vi "UHR-Fleezers Control (host) -Leonardo 04-2018 V4_fish.vi"(0 "Tab Green FB":T5(tab)=enum."Trap Control (RF)") -> ()   [LabVIEW 2014] (continued)
                n1375 = Divide "Y V/pix"(x=w2136, y=w2151) -> (x/y=w2150:dbl)
                n1376 = Divide "Y half step offset"(x=w2136, y=2.0) -> (x/y=w2152:dbl)
                n1377 = Divide "X pix/step"(x=w2140, y=w2143) -> (x/y=w2149:dbl)
                n1378 = Negate(x=w2152) -> (-x=w2153:dbl)
                n1379 = local read "Initial Y"() -> (w2159:dbl)
                n1380 = Multiply(x=w2141, y=w2150) -> (x*y=w2160:dbl)
                n1381 = Divide "X half step offset"(x=w2136, y=2.0) -> (x/y=w2146:dbl)
                n1382 = Divide "X V/pix"(x=w2136, y=w2149) -> (x/y=w2148:dbl)
                n1383 = Multiply(x=w2136, y=w2143) -> (x*y=w2155:dbl)
                n1384 = Compound Arithmetic op=ADD(w2153, w2160, w2159) -> (w2137:dbl)
                "Pointer Y (V)" <- w2137
                n1385 = Multiply(x=w2148, y=w2142) -> (x*y=w2157:dbl)
                n1386 = Negate(x=w2146) -> (-x=w2145:dbl)
                n1387 = local read "Initial X"() -> (w2158:dbl)
                n1388 = Negate(x=w2157) -> (-x=w2156:dbl)
                n1389 = Compound Arithmetic op=ADD(w2145, w2155, w2158, w2156) -> (w2138:dbl)
                "Pointer X (V)" <- w2138
                n1390 = Or(x="Set X Only", y="Set Confocal Spot (X-Y)") -> (x .or. y?=w2131:bool)
                n1391 = Or(x="Set Confocal Spot (X-Y)", y="Set Y Only") -> (x .or. y?=w2130:bool)
                n1392 = case shown="True" w2131 {
                  tunnel: w2138 -> [_ w2161]
                  frame False {
                  }
                  frame True {
                    n1393 = property on="AO2" class="Slide (strict)"("Val(Sgnl)"=w2161) -> ()  [unwired: 2 in, 2 out]
                  }
                }
                n1394 = case shown="True" w2130 {
                  tunnel: w2137 -> [_ w2162]
                  frame False {
                  }
                  frame True {
                    n1395 = property on="AO1" class="Slide (strict)"("Val(Sgnl)"=w2162) -> ()  [unwired: 2 in, 2 out]
                  }
                }
                n1396 = local write "Set Confocal Spot (X-Y)"(w2135) -> ()
                n1397 = local write "Set X Only"(w2135) -> ()
                n1398 = local write "Set Y Only"(w2135) -> ()
              }
            }
          }
          frame 3 {
            n1399 = local read "BD 2 Frequency 1 (MHz)"() -> (w2163:dbl)
            n1400 = local read "BD 1 Frequency 1 (MHz)"() -> (w2164:dbl)
            n1401 = local write "Manipulating Trap"(TRUE ("Manipulating Trap")) -> ()
            n1402 = local write "Coords"(T8 {"Horizontal"=0, "Vertical"=0} ("Coords")) -> ()
            n1403 = while {
              tunnel: w2169 -> [w2174]
              tunnel: w2167 -> [w2173]
              tunnel: w2165 -> [w2172]
              tunnel: w2164 -> [w2171]
              tunnel: w2163 -> [w2170]
              stop <- w2175 stop-if-true
              n1404 = event shown="[0] \"Pane\": Mouse Move" {
                selector: _ -> [_ _]
                dyn-events: _ -> [_ _]
                timeout: _ -> [_ _]
                tunnel: ["Force Manip Abort" w2239] -> w2175
                tunnel: w2174 -> [w2182 _]
                tunnel: w2173 -> [w2180 _]
                tunnel: w2172 -> [w2179 _]
                tunnel: w2171 -> [w2178 _]
                tunnel: w2170 -> [w2177 _]
                event Mouse Move {
                  n1405 = event-data() -> ("Time"=w2183:u32, "Coords"=w2184:T8)  [unwired: 3 out]
                  n1406 = Less?(x=w2183, y=w2182) -> (x < y?=w2181:bool)
                  n1407 = case "Makes sure old motion events prior to mouse click aren't used" shown="False" w2181 {
                    tunnel: w2184 -> [w2226 _]
                    tunnel: w2180 -> [w2227 _]
                    tunnel: w2179 -> [w2204 _]
                    tunnel: w2178 -> [w2200 _]
                    tunnel: w2177 -> [w2199 _]
                    frame False {
                      n1408 = Subtract(x=w2226, y=w2227) -> (x-y=w2225:T8)
                      "Coords" <- w2225
                      n1409 = local read "Y RF Frequency Limits (MHz)"() -> (w2185:T16)
                      n1410 = To Double Precision Float(number=w2225) -> (double precision float=w2224:cluster{"Horizontal":dbl, "Vertical":dbl})
                      n1411 = Multiply(x=cluster{"Horizontal":dbl, "Vertical":dbl} {"Horizontal"=-1.0, "Vertical"=1.0}, y="Manipulation Scaling") -> (x*y=w2220:cluster{"Horizontal":dbl, "Vertical":dbl})
                      n1412 = local read "X RF Frequency Limits (MHz)"() -> (w2186:T16)
                      n1413 = Multiply(x=w2224, y=w2220) -> (x*y=w2222:cluster{"Horizontal":dbl, "Vertical":dbl})
                      n1414 = Unbundle By Name(w2222) -> ("Horizontal"=w2217:dbl, "Vertical"=w2221:dbl)
                      n1415 = Unbundle By Name(w2185) -> ("Maximum"=w2188:dbl, "Minimum"=w2187:dbl)
                      n1416 = Boolean To (0,1)(Boolean="Manip. X?") -> (0, 1=w2215:i16)
                      n1417 = Boolean To (0,1)(Boolean="Manip. Y?") -> (0, 1=w2212:i16)
                      n1418 = local read "BD 1 Frequency 2 (MHz)"() -> (w2202:dbl)
                      n1419 = Multiply(x=w2221, y=w2212) -> (x*y=w2214:dbl)
                      n1420 = Multiply(x=w2215, y=w2217) -> (x*y=w2218:dbl)
                      n1421 = local read "BD 2 Frequency 2 (MHz)"() -> (w2201:dbl)
                      n1422 = Unbundle By Name(w2186) -> ("Maximum"=w2190:dbl, "Minimum"=w2189:dbl)
                      n1423 = Add(x=w2199, y=w2214) -> (x+y=w2192:dbl)
                      n1424 = Add(x=w2200, y=w2218) -> (x+y=w2194:dbl)
                      n1425 = In Range and Coerce(upper limit=w2190, x=w2194, lower limit=w2189) -> (coerced(x)=w2193:dbl)  [unwired: 1 out]
                      n1426 = In Range and Coerce(upper limit=w2188, x=w2192, lower limit=w2187) -> (coerced(x)=w2191:dbl)  [unwired: 1 out]
                      n1427 = Subtract(x=w2193, y=w2202) -> (x-y=w2211:dbl)
                      n1428 = Subtract(x=w2191, y=w2201) -> (x-y=w2210:dbl)
                      n1429 = Square(x=w2211) -> (x^2=w2209:dbl)
                      n1430 = Square(x=w2210) -> (x^2=w2208:dbl)
                      n1431 = Add(x=w2209, y=w2208) -> (x+y=w2207:dbl)
                      n1432 = Square Root(x=w2207) -> (sqrt(x)=w2203:dbl)
                      n1433 = In Range and Coerce(upper limit="Limit Max (MHz)", x=w2203, lower limit="Limit Min (MHz)") -> (In Range?=w2196:bool)  [unwired: 1 out]
                      n1434 = Not(x="Limits Enable") -> (.not. x?=w2195:bool)
                      n1435 = Or(x=w2196, y=w2195) -> (x .or. y?=w2197:bool)
                      n1436 = case shown="True" w2197 {
                        tunnel: w2204 -> [_ w2237]
                        tunnel: w2203 -> [_ w2228]
                        tunnel: w2193 -> [_ w2235]
                        tunnel: w2202 -> [_ w2234]
                        tunnel: w2191 -> [_ w2233]
                        tunnel: w2201 -> [_ w2232]
                        tunnel: w2186 -> [_ w2230]
                        tunnel: w2185 -> [_ w2229]
                        frame False {
                        }
                        frame True {
                          n1437 = local read "BD 1 Frequency 3 (MHz)"() -> (w2236:dbl)
                          n1438 = local read "BD 2 Frequency 3 (MHz)"() -> (w2231:dbl)
                          n1439 = local write "Trap Delta (MHz)"(w2228) -> ()
                          n1440 = property on="Initial delta (MHz)" class="DigNum (strict)"("Val(Sgnl)"=w2228) -> ()  [unwired: 2 in, 2 out]
                          n1441 = call "set RF board frequency - interlace.vi"("Board 2 Frequency Limits"=w2229, "Board 1 Frequency Limits"=w2230, "FPGA VI Reference In"=w2237, "Board 2 Frequency 3 (MHz)"=w2231, "Board 1 Frequency 3 (MHz)"=w2236, "Board 2 Frequency 2 (MHz)"=w2232, "Board 2 Frequency 1 (MHz)"=w2233, "Board 1 Frequency 2 (MHz)"=w2234, "Board 1 Frequency 1  (MHz)"=w2235) -> ()  [unwired: 1 in, 2 out]
                          n1442 = local write "BD 2 Frequency 1 (MHz)"(w2233) -> ()
                          n1443 = local write "BD 1 Frequency 1 (MHz)"(w2235) -> ()
                        }
                      }
                    }
                    frame True {
                    }
                  }
                }
                event Mouse Up {
                  n1444 = event-data() -> ("Button"=w2238:u16)  [unwired: 8 out]
                  n1445 = case shown="3" w2238 {
                    tunnel: [FALSE TRUE] -> w2239
                    frame 0, Default {
                    }
                    frame 3 {
                      n1446 = local write "Manipulating Trap"(FALSE ("Manipulating Trap")) -> ()
                    }
                  }
                }
              }
            }
          }
        }
      }
      event Mouse Move {
        n1447 = event-data() -> ()  [unwired: 6 out]
      }
    }
    n1448 = local read "Stop All"() -> (w2060:bool)
    n1449 = node-c288() -> ()  [unwired: 2 out]
  }
  n1450 = node-c288(w54) -> ()  [unwired: 1 out]
  n1451 = node-c288(w103) -> ()  [unwired: 1 out]
  n1452 = node-c288(w110) -> ()  [unwired: 1 out]
  n1453 = node-c288(i64 1 ("Period"), 1 ("Processor")) -> (w196:T25)  [unwired: 2 out]
  n1454 = timed-loop "Acquire Data" {
    tunnel: w62 -> [w2550]
    tunnel: w77 -> [w2549]
    tunnel: [w2580] -> w70
    tunnel: [w2574] -> w3
    timing: w196 -> [_]
    timing-out: [_] -> w195
    tunnel: w94 -> [w2396]
    stop <- "Stop All" stop-if-true
    (unwired) u32 0 ("Number of Elements")
    w2383 = "NI_ChannelName" ("name")
    n1455 = node-c288() -> ()  [unwired: 2 out]
    n1456 = First Call?() -> (First Call?: T/F=w2349:bool)
    n1457 = Or(x="Reset", y=w2349) -> (x .or. y?=w2350:bool)
    n1458 = local read "MCL Tracking"() -> (w2287:bool)
    n1459 = case "Reset data stream" shown="True" w2350 {
      tunnel: w2550 -> [w2748 w2756]
      tunnel: w2549 -> [w2747 w2755]
      tunnel: [w2748 w2750] -> w2285
      tunnel: [w2747 w2749] -> w2545
      frame False {
      }
      frame True {
        w2753 = TRUE ("AI to FIFO")
        n1460 = local write "Overflow (data lost)"(FALSE ("Overflow (data lost)")) -> ()
        n1461 = call "reset FPGA DMA.vi"("error in"=w2755, "FPGA VI Reference In"=w2756) -> ("error out"=w2751:errorcluster, "FPGA VI Reference Out"=w2752:T20)
        n1462 = xnode "Read/Write Control"("FPGA VI Reference In"=w2752, "error in"=w2751, "AI to FIFO"=w2753, "APD to FIFO"=w2753) -> ("FPGA VI Reference Out"=w2750:T20, "error out"=w2749:errorcluster)
      }
    }
    n1463 = Or(x="Start AOD Scan", y="Trap Raster Scan") -> (x .or. y?=w2503:bool)
    n1464 = case "Start AOM raster scan" shown="True" w2503 {
      tunnel: w2285 -> [w3489 w3500]
      tunnel: w2545 -> [w3488 w3499]
      tunnel: [w3489 w3493] -> w2284
      tunnel: [w3488 w3492] -> w2544
      frame False {
      }
      frame True {
        n1465 = case shown="True" "Restart DMA? (AOD)" {
          tunnel: [w3540 w3542] -> w3494
          tunnel: [w3539 w3541] -> w3495
          tunnel: w3500 -> [w3540 w3544]
          tunnel: w3499 -> [w3539 w3543]
          frame False {
          }
          frame True {
            n1466 = local write "Overflow (data lost)"(FALSE ("Overflow (data lost)")) -> ()
            n1467 = call "reset FPGA DMA.vi"("error in"=w3543, "FPGA VI Reference In"=w3544) -> ("error out"=w3541:errorcluster, "FPGA VI Reference Out"=w3542:T20)
          }
        }
        n1468 = local write "Trap Raster Scan"(FALSE ("Trap Raster Scan")) -> ()
        n1469 = case shown="False" "Move MCL Also?" {
          tunnel: w3495 -> [w3504 w3534]
          tunnel: w3494 -> [w3505 w3535]
          tunnel: [w3503 w3538] -> w3493
          tunnel: [w3502 w3537] -> w3492
          tunnel: "Raster to target force?" -> [w3501 w3507]
          frame False {
            w3506 = TRUE ("AI to FIFO")
            n1470 = xnode "Read/Write Control"("FPGA VI Reference In"=w3505, "error in"=w3504, "AI to FIFO"=w3506, "APD to FIFO"=w3506, "Start scan"=w3506, "Raster to target force"=w3501) -> ("FPGA VI Reference Out"=w3503:T20, "error out"=w3502:errorcluster)
          }
          frame True {
            w3531 = FALSE ("1D or 2D Scan?")
            w3536 = TRUE ("AI to FIFO")
            # "Count for MCL loop"
            # "N total cycles"
            # "N steps"
            # "V_int"
            n1471 = local read "Scan Range (nm)"() -> (w3513:dbl)
            n1472 = local read "Number of F/B Scans (AOD)"() -> (w3530:u16)
            n1473 = Sign(1:w3513) -> (0:w3512:dbl)
            n1474 = Compound Arithmetic op=MULTIPLY(w3513, "MCL Step Position Ratio", "MCL/AOM Scale Tweak") -> (w3517:dbl)
            n1475 = Negate(x=w3512) -> (-x=w3509:dbl)
            n1476 = Multiply(x=w3509, y="MCL Step Increment (V_int)") -> (x*y=w3511:dbl)
            n1477 = Divide(x=w3517, y="MCL X Cal (nm/V)") -> (x/y=w3523:dbl)
            n1478 = Multiply(x=32767.0 ("y"), y=w3523) -> (x*y=w3529:dbl)
            n1479 = local read "Total Counts (ticks)"() -> (w3514:u32)
            n1480 = local read "Cycles/step (AOD)"() -> (w3525:u64)
            n1481 = local read "Scan steps (AOD)"() -> (w3526:u64)
            n1482 = Divide(x=w3529, y=10.0) -> (x/y=w3522:dbl)
            n1483 = Divide(x=w3522, y="MCL Step Increment (V_int)") -> (x/y=w3520:dbl)
            n1484 = Absolute Value(x=w3520) -> (abs(x)=w3508:dbl)
            n1485 = Compound Arithmetic op=MULTIPLY(w3526, w3525, w3514) -> (w3521:u64)
            n1486 = local write "wait to reset values"(w3536) -> ()
            n1487 = local write "MCL Scanning"(w3536) -> ()
            n1488 = Divide(x=w3521, y=w3508) -> (x/y=w3518:dbl)
            "MCL Count" <- w3518
            n1489 = xnode "Read/Write Control"("FPGA VI Reference In"=w3535, "error in"=w3534, "Scan steps (MCL)"=w3508, "Number of scans (MCL)"=w3530, "Cycles per step (MCL)"=u64 1, "Scan freq.  increment (MCL)"=w3511, "1D or 2D Scan?"=w3531, "MCL Scan Axis"=w3531, "Cont. Scan (MCL)"=w3531, "MCL count"=w3518) -> ("FPGA VI Reference Out"=w3533:T20, "error out"=w3532:errorcluster)
            n1490 = xnode "Read/Write Control"("FPGA VI Reference In"=w3533, "error in"=w3532, "AI to FIFO"=w3536, "APD to FIFO"=w3536, "Start scan"=w3536, "Start scan (MCL)"=w3536, "Raster to target force"=w3507) -> ("FPGA VI Reference Out"=w3538:T20, "error out"=w3537:errorcluster)
          }
        }
        "Raster Scanning..." <- TRUE ("Scanning...")
      }
    }
    n1491 = And(x="Save scans", y=w2503) -> (x .and. y?=w2543:bool)
    n1492 = Compound Arithmetic op=OR("Start MCL Scan", "Confocal Image", "Confocal Linescan") -> (w2501:bool)
    n1493 = And(x="Save Data (MCL)", y=w2501) -> (x .and. y?=w2542:bool)
    n1494 = case "Start MCL raster scan" shown="True" w2501 {
      tunnel: w2284 -> [w3039 w3054]
      tunnel: w2544 -> [w3038 w3053]
      tunnel: [w3039 w3049] -> w2319
      tunnel: [w3038 w3048] -> w2318
      tunnel: [FALSE w3047] -> w2528
      tunnel: "Start MCL Scan" -> [_ w3042]
      tunnel: "Confocal Image" -> [_ w3041]
      tunnel: "Confocal Linescan" -> [_ _]
      frame False {
      }
      frame True {
        w3047 = TRUE
        n1495 = case shown="True" "Restart DMA? (MCL)" {
          tunnel: [w3099 w3101] -> w3052
          tunnel: [w3098 w3100] -> w3051
          tunnel: w3054 -> [w3099 w3104]
          tunnel: w3053 -> [w3098 w3103]
          frame False {
          }
          frame True {
            n1496 = call "reset FPGA DMA.vi"("error in"=w3103, "FPGA VI Reference In"=w3104) -> ("error out"=w3100:errorcluster, "FPGA VI Reference Out"=w3101:T20)
            n1497 = local write "Overflow (data lost)"(FALSE ("Overflow (data lost)")) -> ()
          }
        }
        n1498 = case shown="False" w3042 {
          selector: w3042 -> [_ w3058]
          tunnel: w3041 -> [w3057 _]
          tunnel: [w3057 w3058] -> w3040
          frame False {
            n1499 = property on="2D or 1D Scan" class="Bool (strict)"("Val(Sgnl)"=w3057) -> ()  [unwired: 2 in, 2 out]
            n1500 = property on="Confocal Image" class="Bool (strict)"("Value"=FALSE ("Start Confocal Map")) -> ()  [unwired: 2 in, 2 out]
          }
          frame True {
          }
        }
        n1501 = local write "MCL Scanning"(w3047) -> ()
        n1502 = local read "AO1"() -> (w3044:dbl)
        n1503 = local read "AO2"() -> (w3043:dbl)
        n1504 = case shown="True" "Center Scan" {
          tunnel: w3052 -> [w3065 w3097]
          tunnel: w3051 -> [w3064 w3096]
          tunnel: [w3063 w3095] -> w3049
          tunnel: [w3062 w3094] -> w3048
          tunnel: [w3060 w3081] -> w3046
          tunnel: [w3059 w3080] -> w3045
          tunnel: w3044 -> [w3060 w3086]
          tunnel: w3043 -> [w3059 w3089]
          tunnel: w3040 -> [_ _]
          frame False {
            w3061 = TRUE ("AI to FIFO")
            n1505 = xnode "Read/Write Control"("FPGA VI Reference In"=w3065, "error in"=w3064, "AI to FIFO"=w3061, "APD to FIFO"=w3061, "Start scan (MCL)"=w3061) -> ("FPGA VI Reference Out"=w3063:T20, "error out"=w3062:errorcluster)
          }
          frame True {
            w3093 = TRUE ("AI to FIFO")
            n1506 = local read "Scan steps (MCL)"() -> (w3072:u64)
            n1507 = local read "Scan lines (y)"() -> (w3068:u64)
            n1508 = local read "Fast Scan Dir"() -> (w3079:bool)
            n1509 = local read "Actual MCL Inc (V)"() -> (w3069:dbl)
            n1510 = Decrement(x=w3068) -> (x-1=w3067:u64)
            n1511 = Decrement(x=w3072) -> (x-1=w3071:u64)
            n1512 = Multiply(x=w3069, y=w3067) -> (x*y=w3066:dbl)
            n1513 = Divide(x=w3066, y=2.0) -> (x/y=w3076:dbl)
            n1514 = Multiply(x=w3069, y=w3071) -> (x*y=w3070:dbl)
            n1515 = Divide(x=w3070, y=2.0) -> (x/y=w3075:dbl)
            n1516 = Select(t=w3075, s=w3079, f=w3076) -> (s? t:f=w3074:dbl)
            n1517 = Select(t=w3076, s=w3079, f=w3075) -> (s? t:f=w3078:dbl)
            n1518 = Subtract(x=w3086, y=w3078) -> (x-y=w3077:dbl)
            n1519 = Subtract(x=w3089, y=w3074) -> (x-y=w3073:dbl)
            n1520 = local read "2D or 1D Scan"() -> (w3091:bool)
            n1521 = Not(x=w3079) -> (.not. x?=w3085:bool)
            n1522 = Not(x=w3091) -> (.not. x?=w3087:bool)
            n1523 = And(x=w3079, y=w3087) -> (x .and. y?=w3088:bool)
            n1524 = And(x=w3087, y=w3085) -> (x .and. y?=w3090:bool)
            n1525 = Select(t=w3089, s=w3090, f=w3073) -> (s? t:f=w3080:dbl)
            n1526 = Select(t=w3086, s=w3088, f=w3077) -> (s? t:f=w3081:dbl)
            n1527 = call "Volt to I16.vi"("Voltage In"=w3081) -> ("I16 Voltage Out"=w3084:i16)
            n1528 = call "Volt to I16.vi"("Voltage In"=w3080) -> ("I16 Voltage Out"=w3083:i16)
            n1529 = xnode "Read/Write Control"("FPGA VI Reference In"=w3097, "error in"=w3096, "AI to FIFO"=w3093, "APD to FIFO"=w3093, "Start scan (MCL)"=w3093, "AO1 (Y)"=w3084, "AO2 (X)"=w3083) -> ("FPGA VI Reference Out"=w3095:T20, "error out"=w3094:errorcluster)
          }
        }
        "Initial Y" <- w3046
        "Initial X" <- w3045
        "wait to reset values" <- w3047
      }
    }
    n1530 = local read "Trap Pos Elements/DMA read"() -> (w2392:u32)
    n1531 = local read "Trap AI Elements/DMA read"() -> (w2317:u32)
    n1532 = local read "APD Elements/DMA read"() -> (w2431:u32)
    n1533 = local read "Trap AI FIFO Depth"() -> (w2590:u32)
    n1534 = xnode "Invoke Method"("FPGA VI Reference In"=w2319, "error in"=w2318, "Number of Elements"=w2392, "Timeout (ms)"=-1) -> ("Data"=w2356:u16[], "Elements Remaining"=→"Trap Pos FIFO El Remaining":u32)  [unwired: 2 out]
    n1535 = xnode "Invoke Method"("FPGA VI Reference In"=w2319, "error in"=w2318, "Number of Elements"=w2317, "Timeout (ms)"=-1 ("Timeout")) -> ("FPGA VI Reference Out"=w2288:T20, "error out"=w2320:errorcluster, "Data"=w2316:i16[], "Elements Remaining"=w2321:u32)
    "Trap AI FIFO El. Rem." <- w2321
    n1536 = xnode "Get APD Data"("FPGA VI Reference In"=w2319, "error in"=w2318, "Number of Elements"=w2431, "Timeout (ms)"=-1) -> ("Data"=w2430:u32[], "Elements Remaining"=→"APD FIFO Elements Remaining":u32)  [unwired: 2 out]
    n1537 = Subtract(x=w2590, y=w2317) -> (x-y=w2589:u32)
    n1538 = Decimate 1D Array(w2356) -> (w2353:u16[], w2355:u16[], w2354:u16[])
    n1539 = Divide(x=w2321, y=w2589) -> (x/y=w2588:dbl)
    "Buffer Status" <- w2588
    n1540 = To Unsigned Long Integer(number=w2353) -> (unsigned 32bit integer=w2352:u32[])
    n1541 = Join Numbers(hi=w2355, lo=w2354) -> ((hi.lo)=w2351:u32[])
    n1542 = Equal?(x=w2588, y=1.0) -> (x = y?=w2586:bool)
    n1543 = Join Numbers(hi=w2352, lo=w2351) -> ((hi.lo)=w2345:u64[])
    n1544 = call "IR AOM word to freq - vec.vi"("Frequency Word In (double vec)"=w2345) -> ("Frequency Out"=w2391:dbl[])
    n1545 = case "Alert buffer overflow" shown="True" w2586 {
      frame False {
      }
      frame True {
        n1546 = call <vilib>:"Beep.vi"() -> ()  [unwired: 3 in, 9 out]
        "Overflow (data lost)" <- TRUE ("Overflow (data lost)")
      }
    }
    n1547 = Decimate 1D Array(w2391) -> (w2390:dbl[], w2389:dbl[])
    n1548 = Array Size(array=w2316) -> (size(s)=→"Waveform Chart":i32)
    n1549 = Build Array(w2390, w2389) -> (w2388:dbl[][])
    n1550 = local read "Trap Sets"() -> (w2463:u32)
    n1551 = case "Deinterlace trap data, average down PSD" shown="2" w2463 {
      tunnel: w2316 -> [w3134 w3199]
      tunnel: [w3131 w3196] -> w2456
      tunnel: [w3134 w3198] -> w2348
      tunnel: "Detector Type" -> [w3133 w3194]
      tunnel: [w3132 w3197] -> w2455
      tunnel: [w3130 w3195] -> w2561
      frame 1, Default {
        n1552 = Divide(x=w3134, y=3276.7) -> (x/y=w3135:dbl[])
        n1553 = Decimate 1D Array(w3135) -> (w3144:dbl[], w3143:dbl[], w3142:dbl[], w3141:dbl[], w3140:dbl[], w3139:dbl[], w3138:dbl[], w3137:dbl[])
        n1554 = case shown="\"IR-QPD + PSD + FB-QPD position\"" w3133 {
          tunnel: w3144 -> [w3168 w3193]
          tunnel: w3143 -> [w3167 w3192]
          tunnel: w3142 -> [w3152 w3170]
          tunnel: w3141 -> [w3153 w3180]
          tunnel: w3140 -> [w3166 w3191]
          tunnel: w3139 -> [w3165 w3190]
          tunnel: w3138 -> [w3149 w3171]
          tunnel: w3137 -> [w3148 w3169]
          tunnel: [w3147 w3177] -> w3132
          tunnel: [w3146 w3176] -> w3131
          tunnel: [w3145 w3175] -> w3130
          frame "IR-QPD + PSD + FB-QPD", Default {
            w3145 = 0  # Channel pattern
            n1555 = Divide(x=w3168, y=w3153) -> (x/y=w3155:dbl[])
            n1556 = Divide(x=w3167, y=w3153) -> (x/y=w3154:dbl[])
            n1557 = Divide(x=w3166, y=w3149) -> (x/y=w3151:dbl[])
            n1558 = Divide(x=w3165, y=w3148) -> (x/y=w3150:dbl[])
            n1559 = Build Array(w3155, w3154, w3153, w3152, w3151, w3150, w3149, w3148) -> (w3146:dbl[][])
            n1560 = Bundle("T1 Y", "T1 X", "T1 Sum", "FB Sum", "PSD Y", "PSD X", "PSD Y Sum", "PSD X Sum") -> (w3164:T42)  [unwired: 1 out]
            n1561 = Cluster To Array(cluster=w3164) -> (array=w3147:string[])
          }
          frame "IR-QPD + PSD + FB-QPD position" {
            w3175 = 3  # Channel pattern
            n1562 = Negate(x=w3171) -> (-x=w3172:dbl[])
            n1563 = Divide(x=w3193, y=w3180) -> (x/y=w3182:dbl[])
            n1564 = Divide(x=w3192, y=w3180) -> (x/y=w3181:dbl[])
            n1565 = Divide(x=w3191, y=w3171) -> (x/y=w3179:dbl[])
            n1566 = Divide(x=w3190, y=w3172) -> (x/y=w3178:dbl[])
            n1567 = Build Array(w3182, w3181, w3180, w3169, w3170, w3179, w3178, w3171) -> (w3176:dbl[][])
            n1568 = Bundle("T1 Y", "T1 X", "T1 Sum", "FB X", "FB Sum", "PSD Y", "PSD X", "PSD Y Sum") -> (w3189:T42)  [unwired: 1 out]
            n1569 = Cluster To Array(cluster=w3189) -> (array=w3177:string[])
          }
        }
      }
      frame 2 {
        n1570 = case shown="\"UCB Fleezers 052511\"" w3194 {
          tunnel: w3199 -> [w3261 w3328 w3367 w3467]
          tunnel: [w3200 w3320 w3363 w3398] -> w3198
          tunnel: [w3227 w3311 w3365 w3445] -> w3197
          tunnel: [w3226 w3275 w3356 w3412] -> w3196
          tunnel: [w3220 w3310 w3397 w3443] -> w3195
          frame "IR-QPD + PSD + FB-QPD", Default {
            w3220 = 1  # Channel pattern
            # "time average x2 the 4th signal and the 4 psd signals (detection laser)"
            # "deinterlace 3 signals from qpd"
            n1571 = Decimate 1D Array(w3261) -> (w3260:i16[], w3259:i16[], w3225:i16[], w3258:i16[], w3248:i16[], w3246:i16[], w3245:i16[], w3243:i16[])
            n1572 = call "downsample 1D array - double.vi"("Ave N"=2.0, "Array In"=w3248) -> ("Array Out"=w3247:dbl[])  [unwired: 1 out]
            n1573 = call "downsample 1D array - double.vi"("Ave N"=2.0, "Array In"=w3243) -> ("Array Out"=w3242:dbl[])  [unwired: 1 out]
            n1574 = call "downsample 1D array - double.vi"("Ave N"=2.0, "Array In"=w3245) -> ("Array Out"=w3244:dbl[])  [unwired: 1 out]
            n1575 = call "downsample 1D array - double.vi"("Ave N"=2.0, "Array In"=w3246) -> ("Array Out"=w3228:dbl[])  [unwired: 1 out]
            n1576 = Decimate 1D Array(w3260) -> (w3257:i16[], w3229:i16[])
            n1577 = Decimate 1D Array(w3259) -> (w3256:i16[], w3254:i16[])
            n1578 = Decimate 1D Array(w3258) -> (w3255:i16[], w3253:i16[])
            n1579 = Decimate 1D Array(w3225) -> (w3224:i16[], w3223:i16[])
            n1580 = Interleave 1D Arrays(w3257, w3256, w3255, w3229, w3254, w3253, w3224, w3223, w3247, w3228, w3244, w3242) -> (w3241:dbl[])
            n1581 = To Word Integer(number=w3241) -> (16bit integer=w3200:i16[])
            n1582 = Divide(x=w3241, y=3276.7) -> (x/y=w3240:dbl[])
            n1583 = Decimate 1D Array(w3240) -> (w3239:dbl[], w3238:dbl[], w3237:dbl[], w3236:dbl[], w3235:dbl[], w3234:dbl[], w3222:dbl[], w3221:dbl[], w3233:dbl[], w3232:dbl[], w3231:dbl[], w3230:dbl[])
            n1584 = Divide(x=w3239, y=w3237) -> (x/y=w3207:dbl[])
            n1585 = Divide(x=w3238, y=w3237) -> (x/y=w3206:dbl[])
            n1586 = Divide(x=w3236, y=w3234) -> (x/y=w3205:dbl[])
            n1587 = Divide(x=w3235, y=w3234) -> (x/y=w3204:dbl[])
            n1588 = Divide(x=w3233, y=w3231) -> (x/y=w3203:dbl[])
            n1589 = Divide(x=w3232, y=w3230) -> (x/y=w3202:dbl[])
            n1590 = Bundle("T1 Y", "T1 X", "T1 Sum", "T2 Y", "T2 X", "T2 Sum", "T1 FB Sum", "T2 FB Sum", "PSD Y", "PSD X", "PSD Y Sum", "PSD X Sum") -> (w3208:T43)  [unwired: 1 out]
            n1591 = Build Array(w3207, w3206, w3237, w3205, w3204, w3234, w3222, w3221, w3203, w3202, w3231, w3230) -> (w3226:dbl[][])
            n1592 = Cluster To Array(cluster=w3208) -> (array=w3227:string[])
          }
          frame "IR-QPD + PSD + FB-QPD X position" {
            w3310 = 2  # Channel pattern
            # "convert\nADC numbers\nto volts"
            # "time average x2 the 3 psd signals (detection laser)"
            # "deinterlace 3 signals from qpds"
            n1593 = Decimate 1D Array(w3328) -> (w3327:i16[], w3326:i16[], w3263:i16[], w3264:i16[], w3273:i16[], w3270:i16[], w3267:i16[], w3298:i16[])
            n1594 = Decimate 1D Array(w3327) -> (w3325:i16[], w3312:i16[])
            n1595 = call "downsample 1D array - I16.vi"("Ave N"=2.0, "Array In"=w3273) -> ("Array Out"=w3271:i16[])  [unwired: 1 in]
            n1596 = call "downsample 1D array - I16.vi"("Ave N"=2.0, "Array In"=w3270) -> ("Array Out"=w3268:i16[])  [unwired: 1 in]
            n1597 = Decimate 1D Array(w3326) -> (w3324:i16[], w3322:i16[])
            n1598 = Decimate 1D Array(w3264) -> (w3323:i16[], w3321:i16[])
            n1599 = Decimate 1D Array(w3298) -> (w3297:i16[], w3295:i16[])
            n1600 = Decimate 1D Array(w3263) -> (w3296:i16[], w3294:i16[])
            n1601 = call "downsample 1D array - I16.vi"("Ave N"=2.0, "Array In"=w3267) -> ("Array Out"=w3265:i16[])  [unwired: 1 in]
            n1602 = Interleave 1D Arrays(w3325, w3324, w3323, w3312, w3322, w3321, w3297, w3296, w3295, w3294, w3271, w3268, w3265) -> (w3320:i16[])
            n1603 = Divide(x=w3320, y=3276.7) -> (x/y=w3319:dbl[])
            n1604 = Decimate 1D Array(w3319) -> (w3318:dbl[], w3317:dbl[], w3316:dbl[], w3315:dbl[], w3314:dbl[], w3313:dbl[], w3286:dbl[], w3284:dbl[], w3283:dbl[], w3281:dbl[], w3280:dbl[], w3279:dbl[], w3276:dbl[])
            n1605 = Divide(x=w3318, y=w3316) -> (x/y=w3302:dbl[])
            n1606 = Divide(x=w3317, y=w3316) -> (x/y=w3301:dbl[])
            n1607 = Divide(x=w3315, y=w3313) -> (x/y=w3300:dbl[])
            n1608 = Divide(x=w3314, y=w3313) -> (x/y=w3299:dbl[])
            n1609 = Divide(x=w3286, y=w3284) -> (x/y=w3285:dbl[])
            n1610 = Divide(x=w3283, y=w3281) -> (x/y=w3282:dbl[])
            n1611 = Divide(x=w3280, y=w3276) -> (x/y=w3278:dbl[])
            n1612 = Negate(x=w3276) -> (-x=w3274:dbl[])
            n1613 = Divide(x=w3279, y=w3274) -> (x/y=w3277:dbl[])
            n1614 = Bundle("T1 Y", "T1 X", "T1 Sum", "T2 Y", "T2 X", "T2 Sum", "T1 FB X", "T1 FB Sum", "T2 FB X", "T2 FB Sum", "PSD Y", "PSD X", "PSD Y Sum") -> (w3303:T44)  [unwired: 1 out]
            n1615 = Build Array(w3302, w3301, w3316, w3300, w3299, w3313, w3285, w3284, w3282, w3281, w3278, w3277, w3276) -> (w3275:dbl[][])
            n1616 = Cluster To Array(cluster=w3303) -> (array=w3311:string[])
          }
          frame "UCB Fleezers 052511" {
            w3397 = 2  # Channel pattern
            n1617 = Select(t=i16 -1, s="Negate X signals", f=i16 1) -> (s? t:f=w3337:i16)
            n1618 = Decimate 1D Array(w3367) -> (w3338:i16[], w3339:i16[], w3350:i16[], w3366:i16[], w3335:i16[], w3333:i16[], w3331:i16[], w3347:i16[])
            n1619 = Multiply(x=w3337, y=w3339) -> (x*y=w3336:i16[])
            n1620 = Decimate 1D Array(w3338) -> (w3395:i16[], w3385:i16[])
            n1621 = Decimate 1D Array(w3336) -> (w3394:i16[], w3393:i16[])
            n1622 = Decimate 1D Array(w3350) -> (w3344:i16[], w3343:i16[])
            n1623 = Decimate 1D Array(w3366) -> (w3349:i16[], w3348:i16[])
            n1624 = Decimate 1D Array(w3333) -> (w3332:i16[])  [unwired: 1 out]
            n1625 = Decimate 1D Array(w3347) -> (w3346:i16[], w3345:i16[])
            n1626 = Decimate 1D Array(w3331) -> (w3330:i16[])  [unwired: 1 out]
            n1627 = Decimate 1D Array(w3335) -> (w3334:i16[])  [unwired: 1 out]
            n1628 = Interleave 1D Arrays(w3395, w3394, w3349, w3385, w3393, w3348, w3346, w3344, w3345, w3343, w3334, w3332, w3330) -> (w3363:i16[])
            n1629 = Divide(x=w3363, y=3276.7) -> (x/y=w3392:dbl[])
            n1630 = Decimate 1D Array(w3392) -> (w3391:dbl[], w3390:dbl[], w3389:dbl[], w3388:dbl[], w3387:dbl[], w3386:dbl[], w3362:dbl[], w3360:dbl[], w3359:dbl[], w3357:dbl[], w3355:dbl[], w3352:dbl[], w3353:dbl[])
            n1631 = Divide(x=w3391, y=w3389) -> (x/y=w3372:dbl[])
            n1632 = Divide(x=w3390, y=w3389) -> (x/y=w3371:dbl[])
            n1633 = Divide(x=w3388, y=w3386) -> (x/y=w3370:dbl[])
            n1634 = Divide(x=w3387, y=w3386) -> (x/y=w3369:dbl[])
            n1635 = Divide(x=w3362, y=w3360) -> (x/y=w3361:dbl[])
            n1636 = Divide(x=w3359, y=w3357) -> (x/y=w3358:dbl[])
            n1637 = Divide(x=w3355, y=w3353) -> (x/y=w3354:dbl[])
            n1638 = Divide(x=w3352, y=w3353) -> (x/y=w3351:dbl[])
            n1639 = Build Array(w3372, w3371, w3389, w3370, w3369, w3386, w3361, w3360, w3358, w3357, w3354, w3351, w3353) -> (w3356:dbl[][])
            n1640 = Bundle("T1 Y", "T1 X", "T1 Sum", "T2 Y", "T2 X", "T2 Sum", "T1 FB X", "T2 FB Sum", "T2 FB X", "T2 FB Sum", "PSD Y", "PSD X", "PSD Sum") -> (w3373:T44)  [unwired: 1 out]
            n1641 = Cluster To Array(cluster=w3373) -> (array=w3365:string[])
          }
          frame "IR-QPD + PSD + FB-QPD XY positions" {
            w3443 = 4  # Channel pattern
            # "time average x2 the 3 psd signals (detection laser)"
            # "deinterlace 3 signals from qpds"
            n1642 = Decimate 1D Array(w3467) -> (w3466:i16[], w3465:i16[], w3444:i16[], w3464:i16[], w3410:i16[], w3456:i16[], w3455:i16[], w3432:i16[])
            n1643 = Decimate 1D Array "QPD Y"(w3466) -> (w3463:i16[], w3446:i16[])
            n1644 = call "downsample 1D array - double.vi"("Ave N"=2.0, "Array In"=w3456) -> ("Array Out"=w3431:dbl[])  [unwired: 1 out]
            n1645 = call "downsample 1D array - double.vi"("Ave N"=2.0, "Array In"=w3455) -> ("Array Out"=w3430:dbl[])  [unwired: 1 out]
            n1646 = Decimate 1D Array "Feedback Sum"(w3444) -> (w3428:i16[], w3426:i16[])
            n1647 = Decimate 1D Array "Feedback Y"(w3410) -> (w3409:i16[], w3408:i16[])
            n1648 = Decimate 1D Array "Feedback X"(w3432) -> (w3429:i16[], w3427:i16[])
            n1649 = Decimate 1D Array "QPD Sum"(w3464) -> (w3461:i16[], w3459:i16[])
            n1650 = Decimate 1D Array "QPD X"(w3465) -> (w3462:i16[], w3460:i16[])
            n1651 = Interleave 1D Arrays(w3463, w3462, w3461, w3446, w3460, w3459, w3409, w3429, w3428, w3408, w3427, w3426, w3431, w3430) -> (w3454:dbl[])
            n1652 = To Word Integer(number=w3454) -> (16bit integer=w3398:i16[])
            n1653 = Divide(x=w3454, y=3276.7) -> (x/y=w3453:dbl[])
            n1654 = Decimate 1D Array(w3453) -> (w3452:dbl[], w3451:dbl[], w3450:dbl[], w3449:dbl[], w3448:dbl[], w3447:dbl[], w3405:dbl[], w3419:dbl[], w3403:dbl[], w3404:dbl[], w3417:dbl[], w3401:dbl[], w3415:dbl[], w3413:dbl[])
            n1655 = Divide(x=w3452, y=w3450) -> (x/y=w3436:dbl[])
            n1656 = Divide(x=w3451, y=w3450) -> (x/y=w3435:dbl[])
            n1657 = Divide(x=w3449, y=w3447) -> (x/y=w3434:dbl[])
            n1658 = Divide(x=w3448, y=w3447) -> (x/y=w3433:dbl[])
            n1659 = Divide(x=w3405, y=w3403) -> (x/y=w3402:dbl[])
            n1660 = Divide(x=w3419, y=w3403) -> (x/y=w3418:dbl[])
            n1661 = Divide(x=w3404, y=w3401) -> (x/y=w3400:dbl[])
            n1662 = Divide(x=w3417, y=w3401) -> (x/y=w3416:dbl[])
            n1663 = Negate(x=w3413) -> (-x=w3411:dbl[])
            n1664 = Divide(x=w3415, y=w3411) -> (x/y=w3414:dbl[])
            n1665 = Bundle("T1 Y", "T1 X", "T1 Sum", "T2 Y", "T2 X", "T2 Sum", "T1 FB Y", "T1 FB X", "T1 FB Sum", "T2 FB Y", "T2 FB X", "T2 FB Sum", "PSD X", "PSD Y Sum") -> (w3399:T45)  [unwired: 1 out]
            n1666 = Build Array(w3436, w3435, w3450, w3434, w3433, w3447, w3402, w3418, w3403, w3400, w3416, w3401, w3414, w3413) -> (w3412:dbl[][])
            n1667 = Cluster To Array(cluster=w3399) -> (array=w3445:string[])
          }
        }
      }
    }
    "AI labels" <- w2455
    n1668 = xnode "Read/Write Control"("FPGA VI Reference In"=w2288) -> ("FPGA VI Reference Out"=w2281:T20, "BD1 Frequency Out 1"=w2302:u64)  [unwired: 1 in, 1 out]
    n1669 = local read "BD 1 Frequency 2 (MHz)"() -> (w2293:dbl)
    n1670 = To Double Precision Float(number=w2302) -> (double precision float=w2299:dbl)
    n1671 = Multiply(x=49125000.0, y=6.0) -> (x*y=w2298:dbl)
    n1672 = Multiply(x=w2299, y=w2298) -> (x*y=w2296:dbl)
    n1673 = Scale By Power Of 2(n=-48, x=w2296) -> (x*2^n=w2295:dbl)
    n1674 = local read "Dynamic Force FB"() -> (w2292:bool)
    n1675 = local read "Trap Pos. FB ON"() -> (w2291:bool)
    n1676 = Divide(x=w2295, y=1000000.0) -> (x/y=w2286:dbl)
    n1677 = case shown="True" w2287 {
      tunnel: w2286 -> [_ w2725]
      tunnel: w2284 -> [_ w2712]
      frame False {
      }
      frame True {
        n1678 = local read "AOM X Cal (nm/MHz)"() -> (w2722:dbl)
        n1679 = local read "Zero T1 position"() -> (w2724:dbl)
        n1680 = Subtract(x=w2725, y=w2724) -> (x-y=w2723:dbl)
        n1681 = Multiply(x=w2723, y=w2722) -> (x*y=w2721:dbl)
        n1682 = local read "MCL X Cal (nm/V)"() -> (w2718:dbl)
        n1683 = Multiply(x=w2721, y="Tracking factor") -> (x*y=w2719:dbl)
        n1684 = local read "Zero MCL x position"() -> (w2717:dbl)
        n1685 = Divide(x=w2719, y=w2718) -> (x/y=w2716:dbl)
        n1686 = Add(x=w2717, y=w2716) -> (x+y=w2709:dbl)
        "Current MCL (V)" <- w2709
        n1687 = Multiply(x=w2709, y=32767.0) -> (x*y=w2713:dbl)
        n1688 = Divide(x=w2713, y=10.0) -> (x/y=w2710:dbl)
        n1689 = To Word Integer(number=w2710) -> (16bit integer=w2711:i16)
        n1690 = xnode "Read/Write Control"("FPGA VI Reference In"=w2712, "AO2 (X)"=w2711) -> ()  [unwired: 1 in, 2 out]
      }
    }
    n1691 = Subtract(x=w2293, y=w2286) -> (x-y=w2282:dbl)
    "Current deltaFreq" <- w2282
    n1692 = Compound Arithmetic op=AND(w2292, w2291, "Real time offset \ncorrection for setpoint") -> (w2289:bool)
    n1693 = case shown="True" w2289 {
      tunnel: w2282 -> [_ w2728]
      tunnel: w2281 -> [_ w2727]
      frame False {
      }
      frame True {
        n1694 = local read "T1 kappa_x (pN/nm)"() -> (w2736:dbl)
        n1695 = local read "T1 alpha_x (nm/V)"() -> (w2737:dbl)
        n1696 = local read "Negate offset difference"() -> (w2738:bool)
        n1697 = local read "Offset file step size"() -> (w2746:dbl)
        n1698 = Multiply(x="Target Force (pN)", y=2.0) -> (x*y=w2734:dbl)
        n1699 = local read "Setpoint offset\nCorrection values"() -> (w2743:dbl[])
        n1700 = Divide(x=w2728, y=w2746) -> (x/y=w2745:dbl)
        n1701 = Select(t=-1, s=w2738, f=1) -> (s? t:f=w2739:i32)
        n1702 = To Long Integer(number=w2745) -> (32bit integer=w2744:i32)
        n1703 = Multiply(x=w2737, y=w2736) -> (x*y=w2733:dbl)
        n1704 = Divide(x=w2734, y=w2733) -> (x/y=w2732:dbl)
        n1705 = Index Array(array=w2743, index=w2744) -> (element=w2742:dbl)
        n1706 = Multiply(x=w2739, y=w2742) -> (x*y=w2731:dbl)
        n1707 = Add(x=w2732, y=w2731) -> (x+y=w2730:dbl)
        n1708 = To Fixed-Point(number=w2730) -> (fixed-point=w2726:fxp<+/-,16,1>)  [unwired: 1 in]
        "Actual setpoint" <- w2726
        n1709 = xnode "Read/Write Control"("FPGA VI Reference In"=w2727, "Trap Pos. FB SP"=w2726) -> ()  [unwired: 1 in, 2 out]
      }
    }
    n1710 = case shown="True" "Take full offset\n data for display" {
      tunnel: [w2695 w2701] -> w2480
      tunnel: [w2694 w2700] -> w2478
      tunnel: w2282 -> [_ w2707]
      frame False {
        n1711 = Divide(x="T2 offset_x (mV)", y=1000.0) -> (x/y=w2694:dbl)
        n1712 = Divide(x="T1 offset_x (mV)", y=1000.0) -> (x/y=w2695:dbl)
      }
      frame True {
        n1713 = local read "Offset Values"() -> (w2708:T14)
        n1714 = local read "Offset file step size"() -> (w2706:dbl)
        n1715 = Unbundle By Name(w2708) -> ("Trap 1X offset"=w2703:dbl[], "Trap 2X offset"=w2702:dbl[])
        n1716 = Divide(x=w2707, y=w2706) -> (x/y=w2705:dbl)
        n1717 = To Long Integer(number=w2705) -> (32bit integer=w2704:i32)
        n1718 = Index Array(array=w2703, index=w2704) -> (element=w2701:dbl)
        n1719 = Index Array(array=w2702, index=w2704) -> (element=w2700:dbl)
      }
    }
    n1720 = Decimate 1D Array(w2430) -> (w2453:u32[], w2398:u32[])
    n1721 = local read "DMA Update Period (s)"() -> (w2464:dbl)
    n1722 = local read "BD 1 Frequency 2 (MHz)"() -> (w2340:dbl)
    n1723 = local read "BD 1 Frequency 1 (MHz)"() -> (w2341:dbl)
    n1724 = Build Array(w2453, w2398) -> (w2525:u32[][])
    n1725 = local read "Data Period (s)"() -> (w2443:dbl)
    n1726 = Decimate 1D Array(w2348) -> (w2371:i16[], w2370:i16[], w2368:i16[], w2367:i16[])  [unwired: 9 out]
    n1727 = To Double Precision Float(number=w2525) -> (double precision float=w2526:dbl[][])
    n1728 = local read "APD Integration Time (s)"() -> (w2411:dbl)
    n1729 = Divide(x=w2371, y=w2370) -> (x/y=w2372:dbl[])
    n1730 = Divide(x=w2368, y=w2367) -> (x/y=w2369:dbl[])
    n1731 = feedback #1(0.0) -> (w2385:dbl)
    n1732 = Add(x=w2464, y=w2385) -> (x+y=w2563:dbl)
    n1733 = feedback-in #1(w2563) -> ()
    n1734 = local read "AOM X Cal (nm/MHz)"() -> (w2338:dbl)
    n1735 = To Time Stamp(1:w2385) -> (0:w2384:timestamp)
    n1736 = Split 1D Array(array=w2372, index="N El. to Ave.") -> (second subarray=w2375:dbl[])  [unwired: 1 out]
    n1737 = Split 1D Array(array=w2369, index="N El. to Ave.") -> (second subarray=w2374:dbl[])  [unwired: 1 out]
    n1738 = local read "Trap X AI1 (DMA)"() -> (w2373:T13)
    n1739 = Multiply(x=w2443, y="Trap Disp. Downsample") -> (x*y=w2386:dbl)
    "Display Period (s)" <- w2386
    n1740 = Bundle("BD 1 Frequency 1 (MHz)"=w2341, "BD 1 Frequency 2 (MHz)"=w2340) -> (w2342:T46)  [unwired: 1 out]
    n1741 = for "Trap AI" {
      tunnel: [w3129] -> w2557 mode=indexing
      tunnel: w2384 -> [w3119]
      tunnel: "Trap Disp. Downsample" -> [w3127]
      tunnel: w2456 -> [w3125] mode=indexing
      tunnel: w2443 -> [w3124]
      tunnel: w2455 -> [w3123] mode=indexing
      tunnel: w2383 -> [w3122]
      tunnel: [w3121] -> w2422 mode=indexing
      tunnel: w2386 -> [w3120]
      n1742 = Bundle By Name("Y"=w3125, "dt"=w3124) -> (w3126:waveform(dbl))  [unwired: 1 out]
      n1743 = Set Waveform Attribute(5:w3123, 6:w3122, 7:w3126) -> (3:w3121:waveform(dbl))  [unwired: 1 in, 2 out]
      n1744 = call "downsample 1D array - double.vi"("Ave N"=w3127, "Array In"=w3125) -> ("Array Out"=w3128:dbl[])  [unwired: 1 out]
      n1745 = Bundle By Name(cluster=w3121, "t0"=w3119, "Y"=w3128, "dt"=w3120) -> (w3129:waveform(dbl))
    }
    n1746 = call-poly <vilib>:"Mean.vi"("X"=w2374) -> ("mean"=w2362:dbl)  [unwired: 1 out]
    n1747 = call-poly <vilib>:"Mean.vi"("X"=w2375) -> ("mean"=w2363:dbl)  [unwired: 1 out]
    n1748 = Cluster To Array(cluster=w2342) -> (array=w2339:dbl[])
    n1749 = Reciprocal(x=w2386) -> (1/x=→"Trap Disp. Freq. (Hz)":dbl)
    n1750 = local read "Data points/scans (MCL)"() -> (w2537:dbl)
    n1751 = To Fixed-Point(number=w2362) -> (fixed-point=w2360:fxp<+/-,16,1>)  [unwired: 1 in]
    n1752 = To Fixed-Point(number=w2363) -> (fixed-point=w2361:fxp<+/-,16,1>)  [unwired: 1 in]
    n1753 = Bundle("Trap 1 Pos.", "Trap 2 Pos.") -> (w2382:cluster{string, string})  [unwired: 1 out]
    n1754 = Bundle By Name(cluster=w2373, "Set 1"=w2361, "Set 2"=w2360) -> (→"Trap X AI1 (DMA)":T13)
    n1755 = Cluster To Array(cluster=w2382) -> (array=w2379:string[])
    n1756 = for "Trap Position" {
      tunnel: w2388 -> [w2769] mode=indexing
      tunnel: "Trap Disp. Downsample" -> [w2768]
      tunnel: w2386 -> [w2766]
      tunnel: w2384 -> [w2765]
      tunnel: w2383 -> [w2763]
      tunnel: w2379 -> [w2762] mode=indexing
      tunnel: [w2761] -> w2337 mode=indexing
      tunnel: w2339 -> [w2759] mode=indexing
      tunnel: w2338 -> [w2757]
      n1757 = call "downsample 1D array - double.vi"("Ave N"=w2768, "Array In"=w2769) -> ("Array Out"=w2767:dbl[])  [unwired: 1 out]
      n1758 = Subtract(x=w2767, y=w2759) -> (x-y=w2760:dbl[])
      n1759 = Multiply(x=w2757, y=w2760) -> (x*y=w2758:dbl[])
      n1760 = Bundle By Name("Y"=w2758, "dt"=w2766, "t0"=w2765) -> (w2764:waveform(dbl))  [unwired: 1 out]
      n1761 = Set Waveform Attribute(5:w2762, 6:w2763, 7:w2764) -> (3:w2761:waveform(dbl))  [unwired: 1 in, 2 out]
    }
    "Trap Positions" <- w2337
    n1762 = Bundle("APD 1", "APD 2") -> (w2556:cluster{string, string})  [unwired: 1 out]
    n1763 = Cluster To Array(cluster=w2556) -> (array=w2553:string[])
    n1764 = for "APD" {
      tunnel: w2526 -> [w3108] mode=indexing
      tunnel: w2411 -> [w3116]
      tunnel: [w3112] -> w2418 mode=indexing
      tunnel: "APD Disp. Scale" -> [w3113]
      tunnel: w2383 -> [w3111]
      tunnel: w2553 -> [w3110] mode=indexing
      tunnel: "APD Disp. Downsample" -> [w3106]
      tunnel: [w3109] -> w2552
      tunnel: w2384 -> [w3105]
      n1765 = call "integrate 1D array interval - double.vi"("Ave N"=w3106, "Array In"=w3108) -> ("Array Out"=w3107:dbl[])  [unwired: 1 out]
      n1766 = Multiply(x=w3116, y=w3106) -> (x*y=w3109:dbl)
      n1767 = Divide(x=w3107, y=w3113) -> (x/y=w3114:dbl[])
      n1768 = Bundle By Name("t0"=w3105, "Y"=w3114, "dt"=w3109) -> (w3115:waveform(dbl))  [unwired: 1 out]
      n1769 = Set Waveform Attribute(5:w3110, 6:w3111, 7:w3115) -> (3:w3112:waveform(dbl))  [unwired: 1 in, 2 out]
    }
    "APD Display Period (s)" <- w2552
    n1770 = Reciprocal(x=w2552) -> (1/x=→"APD Display Freq. (Hz)":dbl)
    n1771 = local read "Display Period (s)"() -> (w2442:dbl)
    n1772 = Increment(x=w2537) -> (x+1=w2538:dbl)
    n1773 = Index Array(array=w2337, index=0) -> (element=w2335:waveform(dbl))
    n1774 = To Double Precision Float(number=w2453) -> (double precision float=w2452:dbl[])
    n1775 = feedback #2(w2538) -> (w2541:dbl)
    n1776 = Select(t=0, s=w2528, f=w2541) -> (s? t:f=w2534:dbl)
    n1777 = Array Size(array=w2452) -> (size(s)=w2540:i32)
    n1778 = Add(x=w2540, y=w2534) -> (x+y=w2535:dbl)
    n1779 = Unbundle By Name(w2335) -> ("Y"=w2333:dbl[])
    n1780 = feedback #3(w2453) -> (w2524:u32[])
    n1781 = Build Array (concatenate)(w2524, w2453) -> (w2521:u32[])
    n1782 = feedback #4(w2398) -> (w2417:u32[])
    n1783 = Divide(x="Bead Sep. Int. Time (s)", y=w2442) -> (x/y=w2331:dbl)
    n1784 = Build Array (concatenate)(w2417, w2398) -> (w2416:u32[])
    n1785 = Greater?(x=w2535, y=w2537) -> (0:w2536:bool)
    n1786 = feedback #5(w2333) -> (w2334:dbl[])
    n1787 = Build Array (concatenate)(w2333, w2334) -> (w2332:dbl[])
    n1788 = Select(t=w2534, s=w2536, f=w2535) -> (s? t:f=w2533:dbl)
    n1789 = feedback-in #2(w2533) -> ()
    n1790 = Array Size(array=w2521) -> (size(s)=w2518:i32)
    n1791 = Array Size(array=w2453) -> (size(s)=w2520:i32)
    n1792 = local read "MCL Scanning"() -> (w2531:bool)
    n1793 = local read "APD Integration Time (s)"() -> (w2425:dbl)
    n1794 = Build Array (concatenate)(w2418, w2557) -> (w2420:waveform(dbl)[])
    "All Signals" <- w2420
    n1795 = Split 1D Array(array=w2332, index=w2331) -> (first subarray=w2325:dbl[])  [unwired: 1 out]
    n1796 = feedback-in #5(w2325) -> ()
    n1797 = Multiply(x=w2520, y="APD Ave N") -> (x*y=w2519:dbl)
    n1798 = Greater?(x=w2518, y=w2519) -> (0:w2522:bool)
    n1799 = Not(x=w2536) -> (.not. x?=w2530:bool)
    n1800 = To Double Precision Float(number=w2398) -> (double precision float=w2397:dbl[])
    n1801 = call-poly <vilib>:"Mean.vi"("X"=w2325) -> ("mean"=w2324:dbl)  [unwired: 1 out]
    "Mean T1 Position (nm)" <- w2324
    n1802 = Subtract(x=w2325, y=w2324) -> (x-y=w2330:dbl[])
    n1803 = Square(x=w2330) -> (x^2=w2329:dbl[])
    n1804 = And(x=w2530, y=w2531) -> (x .and. y?=w2532:bool)
    n1805 = call-poly <vilib>:"Mean.vi"("X"=w2329) -> ("mean"=w2328:dbl)  [unwired: 1 out]
    n1806 = case shown="True" w2522 {
      tunnel: w2521 -> [w2889 w2896]
      tunnel: [w2889 w2894] -> w2469
      tunnel: w2519 -> [_ w2891]
      tunnel: w2518 -> [_ w2895]
      tunnel: w2416 -> [w2888 w2893]
      tunnel: [w2888 w2890] -> w2413
      frame False {
      }
      frame True {
        n1807 = Subtract(x=w2895, y=w2891) -> (x-y=w2892:dbl)
        n1808 = Array Subset(array=w2896, index=w2892, length=w2891) -> (w2894:u32[])
        n1809 = Array Subset(array=w2893, index=w2892, length=w2891) -> (w2890:u32[])
      }
    }
    n1810 = feedback-in #3(w2469) -> ()
    n1811 = feedback-in #4(w2413) -> ()
    n1812 = Or(x=w2532, y=w2528) -> (x .or. y?=w2529:bool)
    n1813 = Square Root(x=w2328) -> (sqrt(x)=w2327:dbl)
    n1814 = Equal?(x="Tab Control Display", y=T36."High Res Display") -> (x = y?=w2459:bool)
    n1815 = Multiply(x="APD Disp. Scale", y=w2418) -> (x*y=w2427:waveform(dbl)[])
    n1816 = Multiply(x="APD Disp. Downsample", y=w2425) -> (x*y=w2423:dbl)
    n1817 = Multiply(x=10.0, y=w2327) -> (x*y=→"Trap 1 Position RMS (A)":dbl)
    n1818 = Divide(x=w2427, y=w2423) -> (x/y=w2395:waveform(dbl)[])
    n1819 = Index Array(array=w2395, index=0) -> (element=w2405:waveform(dbl))
    n1820 = case "For computing FFTs for display" shown="True" "Compute FFT" {
      tunnel: w2422 -> [_ w3573]
      frame False {
      }
      frame True {
        n1821 = Build Array("FFT 1 Choice 1", "FFT 1 Choice 2", "FFT 2 Choice 1", "FFT 2 Choice 2") -> (w3566:u16[])
        n1822 = Array Size(array=w3573) -> (size(s)=w3572:i32)
        n1823 = feedback-in #6(w3566) -> ()
        n1824 = feedback #6(u16[] [100, 100, 100, 100]) -> (w3567:u16[])
        n1825 = feedback-in #7("# Spectra to Ave.") -> ()
        n1826 = feedback #7("# Spectra to Ave.") -> (w3564:dbl)
        n1827 = Not Equal?(x="# Spectra to Ave.", y=w3564) -> (x != y?=w3563:bool)
        n1828 = Not Equal?(x=w3566, y=w3567) -> (x != y?=w3565:bool)
        n1829 = feedback #8(1.0) -> (w3550:dbl)
        n1830 = Compound Arithmetic op=OR("Reset FFT", w3565, w3563) -> (w3548:bool)
        n1831 = Select(t=1.0, s=w3548, f=w3550) -> (s? t:f=w3552:dbl)
        n1832 = Greater?(x=w3552, y="# Spectra to Ave.") -> (0:w3571:bool)
        n1833 = Increment(x=w3552) -> (x+1=w3551:dbl)
        n1834 = feedback-in #8(w3551) -> ()
        n1835 = local read "DMA Update Period (s)"() -> (w3546:dbl)
        n1836 = Multiply(x="# Spectra to Ave.", y=w3546) -> (x*y=→"Ave. Time (s)":dbl)
        n1837 = Build Array(cluster{"f0":dbl, "df":dbl, "magnitude":dbl[]} {"f0"=0.0, "df"=0.0, "magnitude"=[]} ("PSD")) -> (w3555:cluster{"f0":dbl, "df":dbl, "magnitude":dbl[]}[])
        n1838 = Build Array(w3555, w3555, w3555, w3555) -> (w3557:T47)
        n1839 = feedback #9(w3557) -> (w3562:T47)
        n1840 = for {
          N: 4 -> [_]
          tunnel: w3566 -> [w3595] mode=indexing
          tunnel: w3573 -> [w3596]
          tunnel: w3572 -> [w3598]
          tunnel: w3548 -> [w3591]
          tunnel: w3571 -> [w3590]
          tunnel: "# Spectra to Ave." -> [w3589]
          tunnel: [w3588] -> w3561 mode=indexing
          tunnel: w3562 -> [w3593] mode=indexing
          tunnel: [w3592] -> w3549 mode=indexing
          tunnel: w3552 -> [w3587]
          n1841 = Less?(x=w3595, y=w3598) -> (x < y?=w3597:bool)
          n1842 = Index Array(array=w3596, index=w3595) -> (element=w3594:waveform(dbl))
          n1843 = case shown="True" w3597 {
            tunnel: w3594 -> [_ w3615]
            tunnel: w3593 -> [w3600 w3613]
            tunnel: [w3600 w3601] -> w3592
            tunnel: w3591 -> [_ w3612]
            tunnel: w3590 -> [_ w3605]
            tunnel: w3589 -> [_ w3604]
            tunnel: [cluster{"f0":dbl, "df":dbl, "magnitude":dbl[]} {"f0"=0.0, "df"=0.0, "magnitude"=[]} ("PSD") w3606] -> w3588
            tunnel: w3587 -> [_ w3603]
            frame False {
            }
            frame True {
              n1844 = call <vilib>:"Std Deviation and Variance.vi"("X"=w3615) -> ("mean"=w3616:dbl)  [unwired: 1 in, 2 out]
              n1845 = Subtract(x=w3615, y=w3616) -> (x-y=w3614:waveform(dbl))
              n1846 = xnode "Spectral Measurements"("Signals"=w3614) -> ("PSD"=w3608:cluster{"f0":dbl, "df":dbl, "magnitude":dbl[]})  [unwired: 1 in, 1 out]
              n1847 = case shown="False" w3612 {
                tunnel: w3613 -> [w3625 _]
                tunnel: [w3621 w3630] -> w3601
                tunnel: w3608 -> [w3624 w3631]
                tunnel: w3605 -> [w3623 _]
                frame False {
                  n1848 = Build Array (concatenate)(w3625, w3624) -> (w3622:cluster{"f0":dbl, "df":dbl, "magnitude":dbl[]}[])
                  n1849 = case shown="True" w3623 {
                    tunnel: w3622 -> [w3626 w3629]
                    tunnel: [w3626 w3627] -> w3621
                    frame False {
                    }
                    frame True {
                      n1850 = Delete From Array(array=w3629, index=0) -> (array with subset deleted=w3627:cluster{"f0":dbl, "df":dbl, "magnitude":dbl[]}[])  [unwired: 1 in, 1 out]
                    }
                  }
                }
                frame True {
                  n1851 = Build Array(w3631) -> (w3630:cluster{"f0":dbl, "df":dbl, "magnitude":dbl[]}[])
                }
              }
              n1852 = for {
                tunnel: w3601 -> [w3620] mode=indexing
                tunnel: [w3619] -> w3611 mode=indexing
                workers-P: _ -> [_]
                n1853 = Unbundle By Name(w3620) -> ("magnitude"=w3619:dbl[])
              }
              n1854 = Transpose 2D Array(2D array=w3611) -> (transposed array=w3610:dbl[][])
              n1855 = for {
                tunnel: w3610 -> [w3618] mode=indexing
                tunnel: [w3617] -> w3609 mode=indexing
                workers-P: _ -> [_]
                n1856 = Add Array Elements(numeric array=w3618) -> (sum=w3617:dbl)
              }
              n1857 = Select(t=w3604, s=w3605, f=w3603) -> (s? t:f=w3602:dbl)
              n1858 = Divide(x=w3609, y=w3602) -> (x/y=w3607:dbl[])
              n1859 = Bundle By Name(cluster=w3608, "magnitude"=w3607) -> (w3606:cluster{"f0":dbl, "df":dbl, "magnitude":dbl[]})
            }
          }
        }
        n1860 = case shown="True" w3548 {
          tunnel: w3549 -> [w3580 w3586]
